vi "Format Index List.vi"(6 "Add Space (T)":bool=TRUE, 11 "Index Array":i32[](array[numeric])) -> (3 "Index List":string)   [LabVIEW 2021, in "Strings.lvlib"]
uses:
  Strings/Strings.lvlib
panel:
  # "from a list of sorted indices, generate a compact string:\n\n1,2,3,4,6,7,8,,10 ==> 1-4,6-8,10"
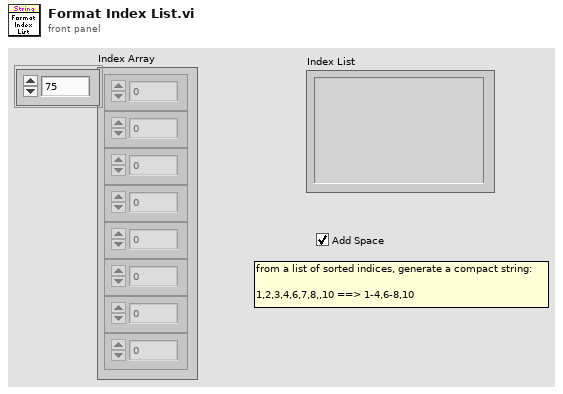
[diagram p1: front panel]
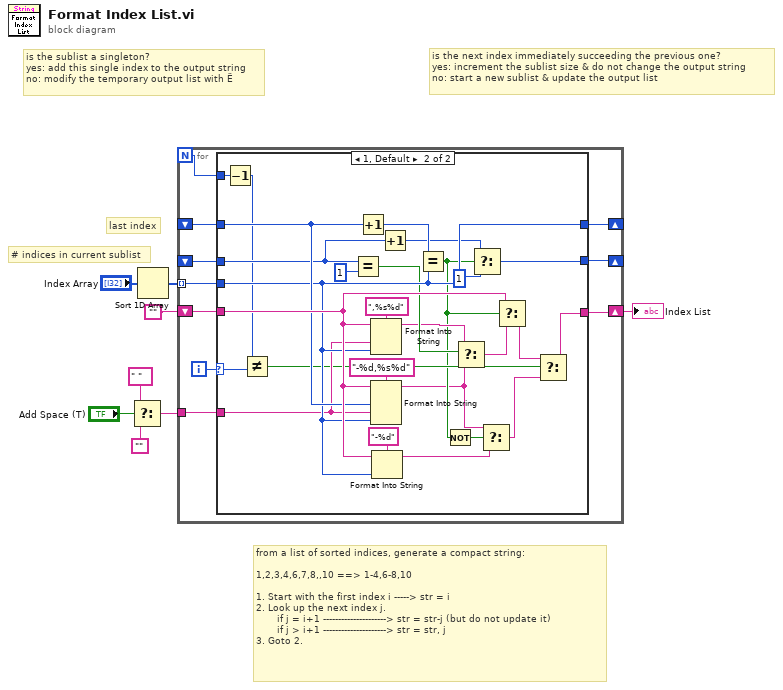
[diagram p0: block diagram]
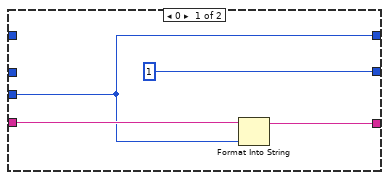
[diagram p2: hidden frame]
diagram:
  # "is the sublist a singleton?\nyes: add this single index to the output string\nno: modify the temporary output list with Ё"
  # "is the next index immediately succeeding the previous one?\nyes: increment the sublist size & do not change the output string\nno: start a new sublist & update the output list"
  # "# indices in current sublist"
  # "last index"
  # "from a list of sorted indices, generate a compact string:\n\n1,2,3,4,6,7,8,,10 ==> 1-4,6-8,10\n\n1. Start with the first index i -----> str = i\n2. Look up the next index j.\n       if j = i+1 ---------------------> str = str-j (but do not update it)\n       if j > i+1 ---------------------> str = str, j\n3. Goto 2."
  n1 = Select(t=" " ("format string"), s="Add Space (T)", f="") -> (s? t:f=w1:string)
  n2 = Sort 1D Array(array="Index Array") -> (sorted array=w7:i32[])
  n3 = for {
    N -> [w9]
    tunnel: w7 -> [w16] mode=indexing
    shift-right: [w17] -> _
    shift-left: _ -> [w13]
    shift-right: [w14] -> w5
    shift-left: "" -> [w15]
    shift-right: [w12] -> _
    shift-left: _ -> [w11]
    tunnel: w1 -> [w10]
    i -> [w18]
    n4 = case shown="1, Default" w18 {
      selector: w18 -> [_ w41]
      tunnel: [w20 w45] -> w17
      tunnel: w16 -> [w20 w45]
      tunnel: w15 -> [w22 w47]
      tunnel: [w21 w49] -> w14
      tunnel: w13 -> [_ w46]
      tunnel: [1 ("Numeric") w48] -> w12
      tunnel: w11 -> [_ w43]
      tunnel: w10 -> [_ w44]
      tunnel: w9 -> [_ w40]
      frame 0 {
        n5 = Format Into String(initial string=w22, w20) -> (resulting string=w21:string)  [unwired: 2 in, 1 out]
      }
      frame 1, Default {
        n6 = Decrement(x=w40) -> (x-1=w39:i32)
        n7 = Not Equal?(x=w39, y=w41) -> (x != y?=w38:bool)
        n8 = Equal?(x=w43, y=1 ("Numeric")) -> (x = y?=w29:bool)
        n9 = Increment(x=w46) -> (x+1=w37:i32)
        n10 = Format Into String(format string=",%s%d", initial string=w47, w44, w45) -> (resulting string=w28:string)  [unwired: 1 in, 1 out]
        n11 = Format Into String(format string="-%d,%s%d", initial string=w47, w46, w44, w45) -> (resulting string=w24:string)  [unwired: 1 in, 1 out]
        n12 = Format Into String(format string="-%d", initial string=w47, w45) -> (resulting string=w42:string)  [unwired: 1 in, 1 out]
        n13 = Increment(x=w43) -> (x+1=w35:i32)
        n14 = Equal?(x=w37, y=w45) -> (x = y?=w25:bool)
        n15 = Not(x=w25) -> (.not. x?=w23:bool)
        n16 = Select(t=w28, s=w29, f=w24) -> (s? t:f=w34:string)
        n17 = Select(t=w35, s=w25, f=1 ("Numeric")) -> (s? t:f=w48:i32)
        n18 = Select(t=w24, s=w23, f=w42) -> (s? t:f=w26:string)
        n19 = Select(t=w47, s=w25, f=w34) -> (s? t:f=w27:string)
        n20 = Select(t=w27, s=w38, f=w26) -> (s? t:f=w49:string)
      }
    }
  }
  "Index List" <- w5
